vi "close.vi"(8 "error in (no error)":errorcluster, 11 "StaticOutputEditor in":refnum<class "StaticOutputEditor.lvclass">) -> (0 "error out":errorcluster, 3 "StaticOutputEditor out":refnum<class "StaticOutputEditor.lvclass">)   [LabVIEW 2009, in "Views.lvlib" / "ScriptEditor.lvlib" / "StaticOutputEditor.lvclass"]
doc: "Close the Static Hardware Front Viewer"
uses:
  StaticOutputEditor.lvclass
  StaticOutputEditor.lvclass/StaticOutputEditor.ctl
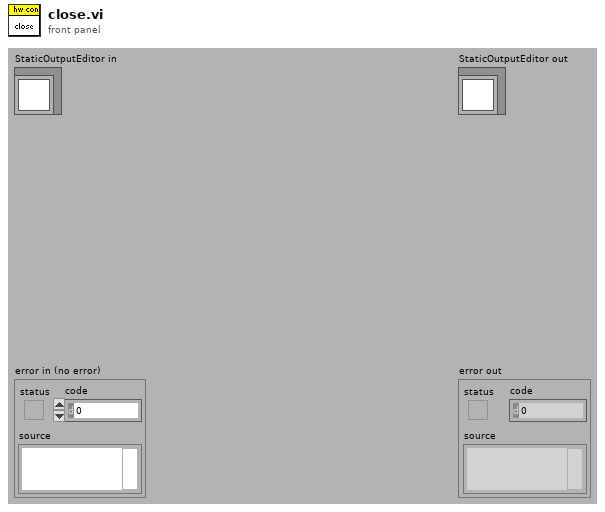
[diagram p1: front panel]
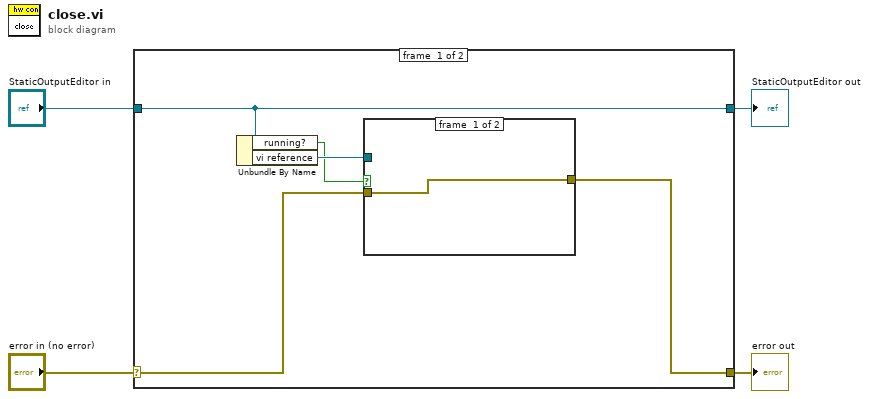
[diagram p0: block diagram]
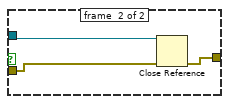
[diagram p2: hidden frame]
diagram:
  n1 = case shown="No Error" "error in (no error)" {
    selector: "error in (no error)" -> [w6 w15]
    tunnel: [w5 w15] -> w3
    tunnel: [w9 w14] -> w1
    tunnel: "StaticOutputEditor in" -> [w9 w14]
    frame #0 {
      n2 = Unbundle By Name(w9) -> ("running?"=w7:bool, "vi reference"=w8:refnum<vi>)
      n3 = case shown="True" w7 {
        tunnel: w8 -> [_ w12]
        tunnel: w6 -> [w10 w11]
        tunnel: [w10 w13] -> w5
        frame #0 {
        }
        frame #1 {
          n4 = Close Reference(reference=w12, error in (no error)=w11) -> (error out=w13:errorcluster)
        }
      }
    }
    frame #1 {
    }
  }
  "error out" <- w3
  "StaticOutputEditor out" <- w1
